vi "Test Queue Synch with passed variable.vi"() -> ()   [LabVIEW 2021]
uses:
  Source/Support/Nodes/abs_Node/Status.ctl
  Source/System/bt_System.lvclass
  Source/Support/Nodes/Decorators/Repeater/Support/Finish On - Type.ctl
  Source/Support/Nodes/Composites/abs_Parallel/Support/Status Calculation.ctl
  Source/Blackboard/Blackboard.lvclass
  Source/Blackboard/Blackboard.lvclass/Blackboard.ctl
  Source/Blackboard/Get Value Type/Get String.vi
  <vilib>/TSA/Abstract Data Classes/Abs_Types/String/Static Write.vi
  <vilib>/TSA/Abstract Data Classes/Abs_Types/String/Static Read.vi
  Source/Blackboard/Support/Index Group.vi
  Source/Blackboard/Support/Index Tags.vi
  <vilib>/TSA/Omni-Bus/Local Bus/Support/STR/Local Bus_String.lvclass
  C:/Program Files (x86)/National Instruments/LabVIEW 2021/vi.lib/TSA/Abstract Data Classes/Abs_Types/Value/Abs_Value.lvclass
  Source/Support/Nodes/Leaves/Synch/Queue/WaitOn/bt_WaitOn_Queue.lvclass
  C:/Users/Tim/Documents/GitHub/LV_Behaviour_Tree/Source/Support/Nodes/abs_Node/bt_Node.lvclass
  Source/Support/Nodes/Leaves/Synch/Queue/Send/bt_Send_Queue.lvclass
  <vilib>/TSA/Omni-Bus/Local Bus/Support/Initialise DVR's.vi
  <vilib>/TSA/Abstract Data Classes/Abs_Types/String/Abs_String.lvclass
  <vilib>/TSA/Abstract Data Classes/Abs_Types/Value/Abs_Value.lvclass
  <vilib>/TSA/Abstract Data Classes/Abs_Types/Type/Abs_Type.lvclass
  <vilib>/TSA/Omni-Bus/Local Bus/Support/DBL/Local Bus_DBL.lvclass
  <vilib>/TSA/Omni-Bus/Local Bus/Support/SGL/Local Bus_SGL.lvclass
  <vilib>/TSA/Omni-Bus/Local Bus/Support/EXT/Local Bus_EXT.lvclass
  <vilib>/TSA/Omni-Bus/Local Bus/Support/Bool/Local Bus_Boolean.lvclass
  <vilib>/TSA/Omni-Bus/Local Bus/Support/Variant/Local Bus_Variant.lvclass
  <vilib>/TSA/Omni-Bus/Local Bus/Support/WFM/Local Bus_Waveform.lvclass
  <vilib>/TSA/Omni-Bus/Local Bus/Support/Time/Local Bus_Time.lvclass
  <vilib>/TSA/Omni-Bus/Local Bus/Support/U8/Local Bus_U8.lvclass
  <vilib>/TSA/Omni-Bus/Local Bus/Support/U16/Local Bus_U16.lvclass
  <vilib>/TSA/Omni-Bus/Local Bus/Support/U32/Local Bus_U32.lvclass
  <vilib>/TSA/Omni-Bus/Local Bus/Support/U64/Local Bus_U64.lvclass
  <vilib>/TSA/Omni-Bus/Local Bus/Support/I8/Local Bus_I8.lvclass
  <vilib>/TSA/Omni-Bus/Local Bus/Support/I16/Local Bus_I16.lvclass
  <vilib>/TSA/Omni-Bus/Local Bus/Support/I32/Local Bus_I32.lvclass
  <vilib>/TSA/Omni-Bus/Local Bus/Support/I64/Local Bus_I64.lvclass
  <vilib>/TSA/Omni-Bus/Local Bus/Support/CSGL/Local Bus_CSGL.lvclass
  <vilib>/TSA/Omni-Bus/Local Bus/Support/CDBL/Local Bus_CDBL.lvclass
  <vilib>/TSA/Omni-Bus/Local Bus/Support/CEXT/Local Bus_CEXT.lvclass
  <vilib>/TSA/Omni-Bus/Local Bus/Support/Type/Local Bus_Type.lvclass
  Source/BT.lvlib
  Source/Support/Nodes/Composites/abs_Parallel/bt_Parallel.lvclass
  Source/Support/Nodes/Decorators/Repeater/bt_Repeater.lvclass
  Source/Support/Nodes/abs_Node/bt_Node.lvclass
panel:
  in  "String 2":string
  out "error out 4":errorcluster
  out "error out 3":errorcluster
  out "error out 2":errorcluster
  out "error out":errorcluster
  out "String":string
  in  "stop":bool
  out "Status":T1
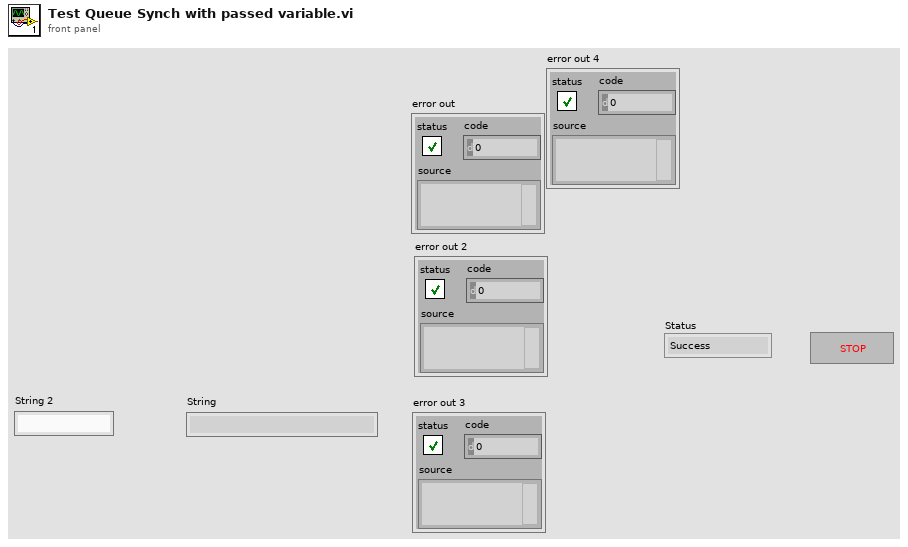
[diagram p1: front panel]
types:
  T1 = typedef "BT.lvlib/bt_Node.lvclass/Status.ctl" = enum16{"Success", "Failure", "Running"}
  T2 = typedef "BT.lvlib/bt_Parallel.lvclass/Status Calculation.ctl" = enum16{"Succeed on All Succeed", "Failure on All Failure", "Succeed on Any Succeed", "Failure on Any Failure"}
  T3 = typedef "BT.lvlib/bt_Repeater.lvclass/Finish On - Type.ctl" = enum16{"Success", "Failure", "Never"}
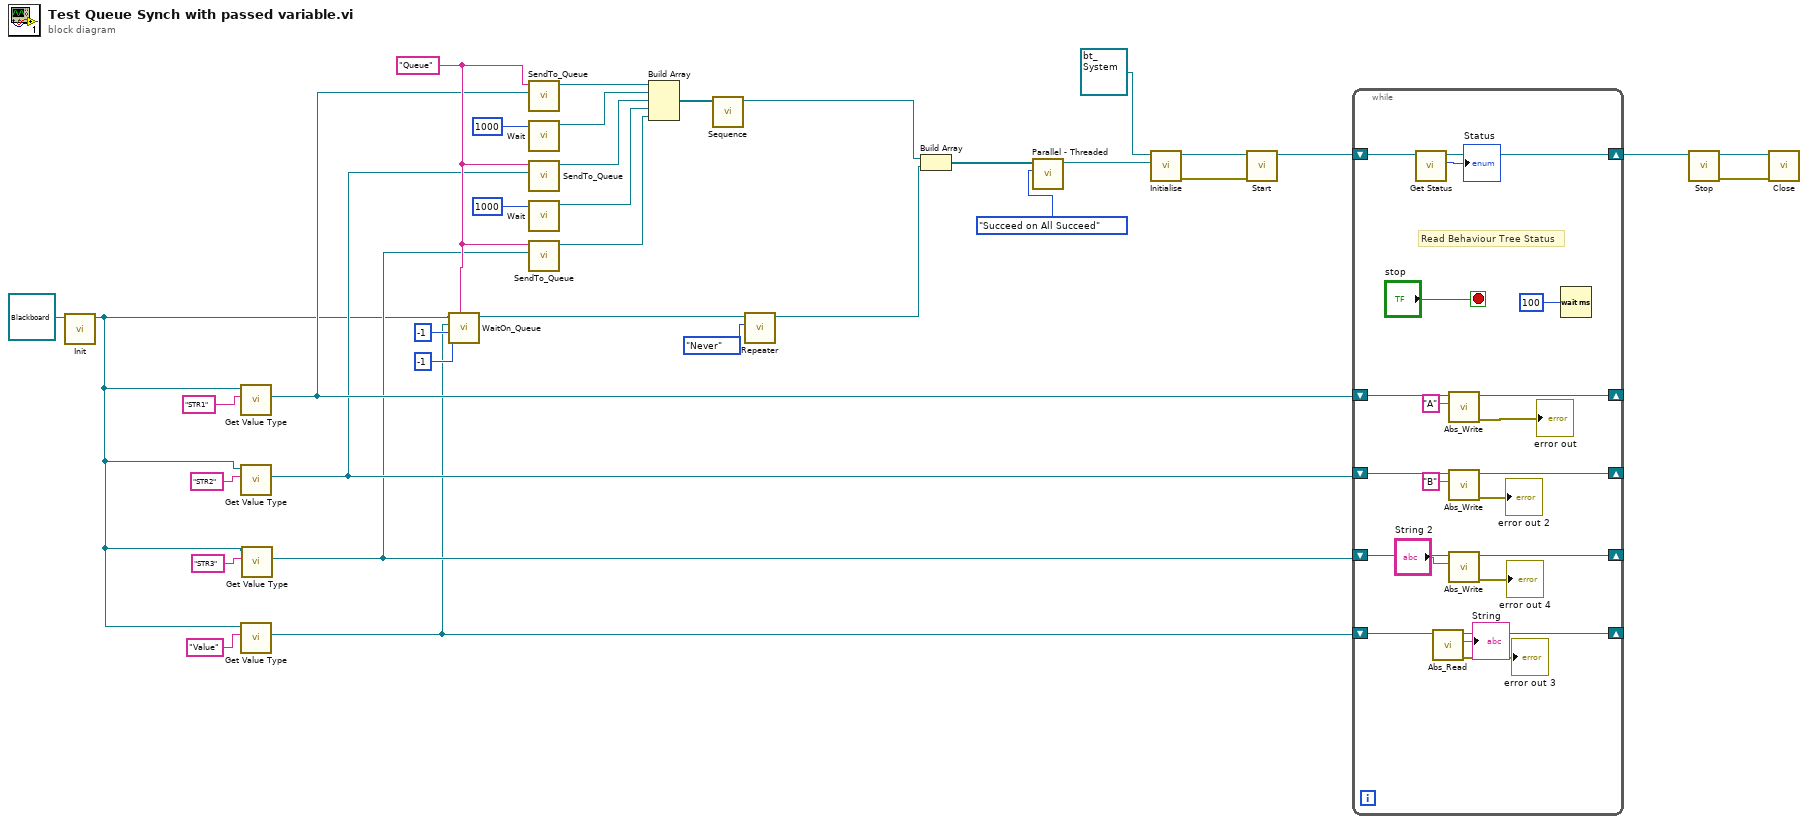
[diagram p0: block diagram]
diagram:
  w7 = "Queue" ("Name")
  n1 = call-dynamic "Init.vi"("bt_Blackboard in"=refnum<class "Blackboard.lvclass"> refnum) -> ("bt_Blackboard out"=w1:refnum<class "Blackboard.lvclass">)  [unwired: 9 in, 1 out]
  n2 = call-poly "Get Value Type.vi"("Tag"="STR1", "Blackboard in"=w1) -> ("Value"=w5:refnum<class "Abs_String.lvclass">)  [unwired: 6 in, 3 out]
  n3 = call-poly "Get Value Type.vi"("Tag"="STR2", "Blackboard in"=w1) -> ("Value"=w4:refnum<class "Abs_String.lvclass">)  [unwired: 6 in, 3 out]
  n4 = call-poly "Get Value Type.vi"("Tag"="Value", "Blackboard in"=w1) -> ("Value"=w2:refnum<class "Abs_String.lvclass">)  [unwired: 6 in, 3 out]
  n5 = call-poly "Get Value Type.vi"("Tag"="STR3", "Blackboard in"=w1) -> ("Value"=w3:refnum<class "Abs_String.lvclass">)  [unwired: 6 in, 3 out]
  n6 = call "WaitOn_Queue.vi"("Queue Name"=w7, "Max Queue Size"=-1, "Timeout (ms)"=-1, "Message Type"=w2, "bt_Blackboard in"=w1) -> ("Queue out"=w19:refnum<class "bt_WaitOn_Queue.lvclass">)  [unwired: 5 in, 1 out]
  n7 = call "SendTo_Queue.vi"("Message"=w5, "Queue Name"=w7) -> ("Queue Out"=w24:refnum<class "bt_Send_Queue.lvclass">)  [unwired: 9 in]
  n8 = call "Wait.vi"("Time (ms)"=u32 1000) -> ("Node Out"=w17:refnum<class "bt_Node.lvclass">)  [unwired: 10 in]
  n9 = call "SendTo_Queue.vi"("Message"=w4, "Queue Name"=w7) -> ("Queue Out"=w22:refnum<class "bt_Send_Queue.lvclass">)  [unwired: 9 in]
  n10 = call "Wait.vi"("Time (ms)"=u32 1000) -> ("Node Out"=w15:refnum<class "bt_Node.lvclass">)  [unwired: 10 in]
  n11 = call "SendTo_Queue.vi"("Message"=w3, "Queue Name"=w7) -> ("Queue Out"=w21:refnum<class "bt_Send_Queue.lvclass">)  [unwired: 9 in]
  n12 = Build Array(w24, w17, w22, w15, w21) -> (w23:refnum<class "bt_Node.lvclass">[])
  n13 = call "Sequence.vi"("Nodes"=w23) -> ("Node"=w20:refnum<class "bt_Node.lvclass">)  [unwired: 10 in]
  n14 = call "Repeater.vi"("Finish On"=Finish_On_-_Type."Never", "Node In"=w19) -> ("Node Out"=w13:refnum<class "bt_Node.lvclass">)  [unwired: 9 in]
  n15 = Build Array(w20, w13) -> (w26:refnum<class "bt_Node.lvclass">[])
  n16 = call "Parallel - Threaded.vi"("Status Calculation"=Status_Calculation."Succeed on All Succeed", "Nodes"=w26) -> ("Node"=w25:refnum<class "bt_Node.lvclass">)  [unwired: 9 in]
  n17 = call "Initialise.vi"("Behaviour Tree"=w25, "bt_System in"=refnum<class "bt_System.lvclass"> refnum) -> ("error out"=w34:errorcluster, "bt_System out"=w35:refnum<class "bt_System.lvclass">)  [unwired: 8 in]
  n18 = call "Start.vi"("error in (no error)"=w34, "bt_System in"=w35) -> ("bt_System out"=w32:refnum<class "bt_System.lvclass">)  [unwired: 8 in, 1 out]
  n19 = while {
    shift-right: [w54] -> w29
    shift-left: w32 -> [w55]
    shift-right: [w50] -> _
    shift-left: w5 -> [w51]
    shift-right: [w48] -> _
    shift-left: w4 -> [w49]
    shift-right: [w46] -> _
    shift-left: w2 -> [w47]
    shift-right: [w40] -> _
    shift-left: w3 -> [w39]
    stop <- "stop" stop-if-true
    # "Read Behaviour Tree Status"
    n20 = call "Get Status.vi"("bt_System in"=w55) -> ("Status"=→"Status":T1, "bt_System out"=w54:refnum<class "bt_System.lvclass">)  [unwired: 8 in, 1 out]
    n21 = call-poly <vilib>:"Abs_Read.vi"("Abs_String in"=w47) -> ("error out"=→"error out 3":errorcluster, "String"=→"String":string, "Abs_String out"=w46:refnum<class "Abs_String.lvclass">)  [unwired: 8 in]
    n22 = call-poly <vilib>:"Abs_Write.vi"("String"="A", "Abs_String in"=w51) -> ("error out"=→"error out":errorcluster, "Abs_String out"=w50:refnum<class "Abs_String.lvclass">)  [unwired: 8 in]
    n23 = call-poly <vilib>:"Abs_Write.vi"("String"="B", "Abs_String in"=w49) -> ("error out"=→"error out 2":errorcluster, "Abs_String out"=w48:refnum<class "Abs_String.lvclass">)  [unwired: 8 in]
    n24 = call-poly <vilib>:"Abs_Write.vi"("String"="String 2", "Abs_String in"=w39) -> ("error out"=→"error out 4":errorcluster, "Abs_String out"=w40:refnum<class "Abs_String.lvclass">)  [unwired: 8 in]
    n25 = Wait (ms)(milliseconds to wait=u32 100) -> ()  [unwired: 1 out]
  }
  n26 = call "Stop.vi"("bt_System in"=w29) -> ("error out"=w30:errorcluster, "bt_System out"=w31:refnum<class "bt_System.lvclass">)  [unwired: 9 in]
  n27 = call-dynamic "Close.vi"("error in (no error)"=w30, "bt_System in"=w31) -> ()  [unwired: 8 in, 2 out]
